vi "2022-BeginCodeOnTarget.vi"(8 "error in":errorcluster) -> (0 "error out":errorcluster)   [LabVIEW 2020]
doc: "Called before other user functions, this VI is expected to open initial I/O refnums, load in file data, and do all program initialization. Notice that the <B>error out</B> terminal is simply used for data flow. Wiring it to other structures or subVIs ensures that this VI runs first."
uses:
  2023LabView/RobV01-NotWorking/Robot Global Data.vi
  <vilib>/Rock Robotics/WPI/DriverStation/WPI_DriverStationRobotMode2.ctl
  <vilib>/Rock Robotics/Network Tables/NT Write String Array.vi
  2022 Robot Global Data.vi
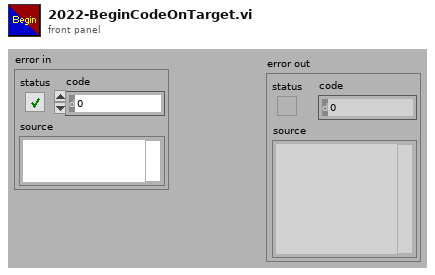
[diagram p1: front panel]
types:
  T1 = typedef "WPI_DriverStationRobotMode2.ctl" = enum16{"Autonomous Disabled", "Autonomous Enabled", "Teleop Disabled", "Teleop Enabled", "Disconnected", "Finish", "Test Disabled", "Test Enabled", "Emergency Stopped"}
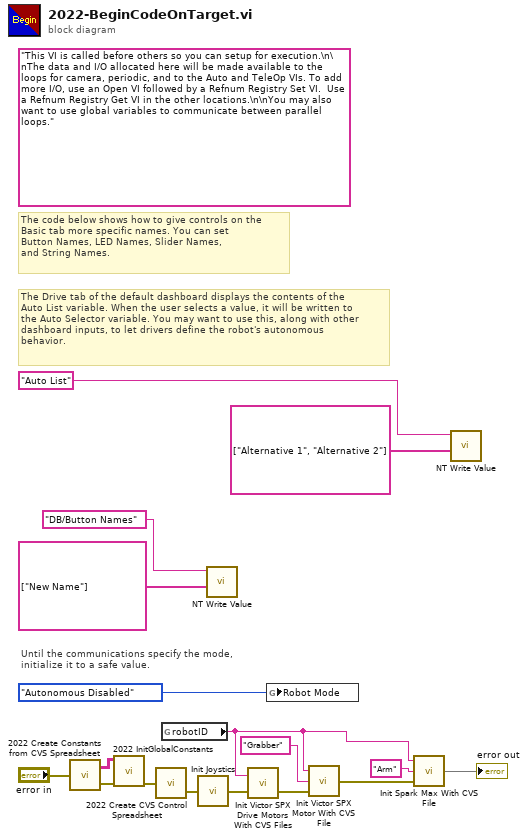
[diagram p0: block diagram]
diagram:
  (unwired) "This VI is called before others so you can setup for execution.\n\nThe data and I/O allocated here will be made available to the loops for camera, periodic, and to the Auto and TeleOp VIs. To add more I/O, use an Open VI followed by a Refnum Registry Set VI.  Use a Refnum Registry Get VI in the other locations.\n\nYou may also want to use global variables to communicate between parallel loops."
  # "The Drive tab of the default dashboard displays the contents of the\nAuto List variable. When the user selects a value, it will be written to\nthe Auto Selector variable. You may want to use this, along with other\ndashboard inputs, to let drivers define the robot's autonomous\nbehavior."
  # "The code below shows how to give controls on the\nBasic tab more specific names. You can set\nButton Names, LED Names, Slider Names,\nand String Names."
  # "Until the communications specify the mode,\ninitialize it to a safe value."
  n1 = call "2022 Create Constants from CVS Spreadsheet.vi"("error in"="error in") -> ("localConstantSpreadSheet"=w11:string[][], "error out"=w10:errorcluster)
  n2 = call "2022 InitGlobalConstants.vi"("error in (no error)"=w10, "localConstantSpreadSheet"=w11) -> ("error out"=w9:errorcluster)  [unwired: 9 in]
  n3 = call "2022 Create CVS Control Spreadsheet.vi"("error in"=w9) -> ("error out"=w8:errorcluster)  [unwired: 1 out]
  n4 = global read "2022 Robot Global Data.vi" "robotID"() -> (w6:string)
  n5 = call "Init Joystics.vi"("error in"=w8) -> ("error out"=w5:errorcluster)
  n6 = call-poly <vilib>:"NT Write Value.vi"("value"=string[] ["New Name"], "name"="DB/Button Names" ("Name")) -> ()  [unwired: 9 in, 1 out]
  n7 = call "Init Victor SPX Drive Motors With CVS Files.vi"("error in"=w5, "Robot ID"=w6) -> ("error out"=w4:errorcluster)  [unwired: 1 out]
  n8 = global write "Robot Global Data.vi" "Robot Mode"(WPI_DriverStationRobotMode2."Autonomous Disabled" ("Robot Mode")) -> ()
  n9 = call "Init Victor SPX Motor With CVS File.vi"("error in"=w4, "Motor ID"="Grabber", "Robot ID"=w6) -> ("error out"=w3:errorcluster)  [unwired: 1 in, 1 out]
  n10 = call "Init Spark Max With CVS File.vi"("error in"=w3, "Motor ID"="Arm", "Robot ID"=w6) -> (1:→"error out")  [unwired: 2 out]
  n11 = call-poly <vilib>:"NT Write Value.vi"("value"=string[] ["Alternative 1", "Alternative 2"] ("String Array"), "name"="Auto List" ("Name")) -> ()  [unwired: 9 in, 1 out]
